vi "ProdaNG.Tree.Test.Update.vi"(5 "Identification":T4, 6 "FileContent":T1, 7 "TreeControl in":refnum<vi>, 8 "error in (no error)":errorcluster, 10 "TreeViewMode (All)":T5, 11 "dbHandle in":i32) -> (0 "error out":errorcluster, 1 "#changes":i32, 2 "Number of Rows":i32, 3 "dbHandle out":i32)   [LabVIEW 2016]
uses:
  ProdaNG.Tree.TestViewMode.ctl
  ProdaNG.File.Sequence.ctl
  ProdaNG.Tree.Fglb.Value.ctl
  ProdaNG.File.Step.ctl
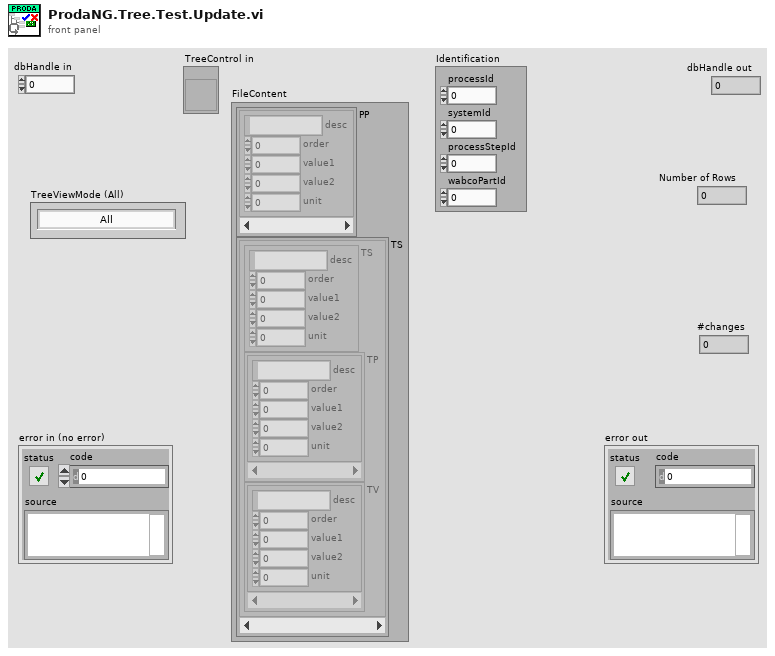
[diagram p1: front panel]
types:
  T1 = typedef "ProdaNG.File.Sequence.ctl" = cluster{"PP":T2[], "TS":T3[]}
  T2 = typedef "ProdaNG.Tree.Fglb.Value.ctl" = cluster{"desc":string, "order":i32, "value1":dbl, "value2":dbl, "unit":i32}
  T3 = typedef "ProdaNG.File.Step.ctl" = cluster{"TS":T2, "TP":T2[], "TV":T2[]}
  T4 = cluster{"processId":i32, "systemId":i32, "processStepId":i32, "wabcoPartId":i32}
  T5 = typedef "ProdaNG.Tree.TestViewMode.ctl" = enum16{"All", "Released", "Unreleased"}
  T6 = typedef "ProdaNG.UnitSimple.ctl" = cluster{"name":string, "i_id":i32}
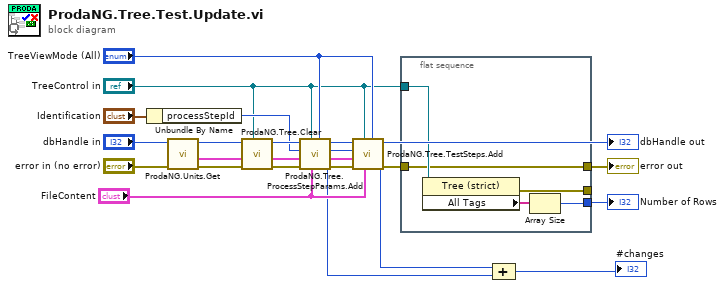
[diagram p0: block diagram]
diagram:
  n1 = Unbundle By Name("Identification") -> ("processStepId"=w17:i32)
  n2 = call "ProdaNG.Units.Get.vi"("error in (no error)"="error in (no error)", "dbHandleIn"="dbHandle in") -> ("error out"=w14:errorcluster, "units simple"=w16:T6[], "dbHandle"=w18:i32)  [unwired: 6 in, 1 out]
  n3 = call "ProdaNG.Tree.Clear.vi"("TestStepsTree"="TreeControl in", "error in (no error)"=w14) -> ("error out"=w15:errorcluster)  [unwired: 9 in]
  n4 = call "ProdaNG.Tree.ProcessStepParams.Add.vi"("Mode"="TreeViewMode (All)", "FileContent"="FileContent", "TestStepsTree"="TreeControl in", "error in (no error)"=w15, "units"=w16, "processStepId"=w17, "dbHandleIn"=w18) -> ("error out"=w10:errorcluster, "#changes"=w2:i32, "dbHandle"=w11:i32)  [unwired: 2 in]
  n5 = call "ProdaNG.Tree.TestSteps.Add.vi"("Mode"="TreeViewMode (All)", "FileContent"="FileContent", "TestStepsTree"="TreeControl in", "error in (no error)"=w10, "units"=w16, "processStepId"=w17, "dbHandleIn"=w11) -> ("error out"=w8:errorcluster, "#changes"=w1:i32, "dbHandle"=→"dbHandle out":i32)  [unwired: 2 in]
  n6 = flat-sequence {
    tunnel: w8 -> [w23]
    tunnel: "TreeControl in" -> [w25]
    tunnel: [w23] -> w6
    tunnel: [w21] -> w5
    tunnel: [w22] -> _
    frame #0 {
      n7 = property class="Tree (strict)"(reference=w25) -> (error out=w22:errorcluster, "All Tags"=w24:string[])  [unwired: 1 in, 1 out]
      n8 = Array Size(array=w24) -> (size(s)=w21:i32)
    }
  }
  n9 = Compound Arithmetic op=ADD(w1, w2) -> (→"#changes":i32)
  "error out" <- w6
  "Number of Rows" <- w5
